vi "Read Disconnected.vi"(8 "error in (no error)":errorcluster, 11 "EventsParent in":refnum<class "Events.lvclass">) -> (0 "error out":errorcluster, 2 "Disconnected":refnum<user-event>, 3 "EventsParent out":refnum<class "Events.lvclass">)   [LabVIEW 2020, in "wamplv.lvlib" / "Events.lvclass"]
uses:
  Events.lvclass
  WAMP Client/API/TypeDefs/Disconnected event data.ctl
  WAMP Client/API/TypeDefs/Termination Reason.ctl
  WAMP Client/Private/TypeDef/Termination Reason Enum.ctl
  Events.lvclass/Events.ctl
  WAMP Client/WAMP Client.lvclass
  wamplv.lvlib
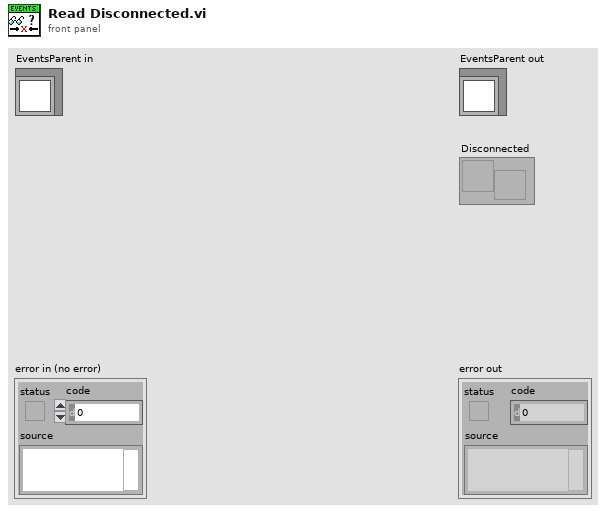
[diagram p1: front panel]
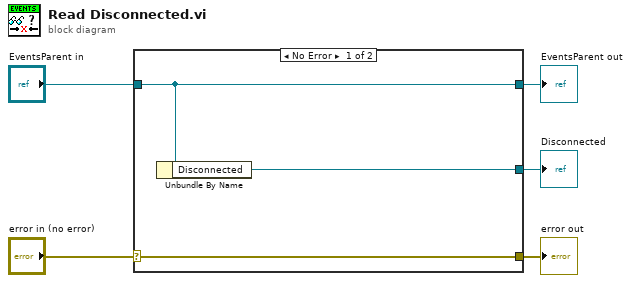
[diagram p0: block diagram]
diagram:
  n1 = case shown="No Error" "error in (no error)" {
    selector: "error in (no error)" -> [w8 w9]
    tunnel: [w8 w9] -> w4
    tunnel: [w7 w10] -> w2
    tunnel: "EventsParent in" -> [w7 w10]
    tunnel: [w6 _] -> w1
    frame No Error {
      n2 = Unbundle By Name(w7) -> ("Disconnected"=w6:refnum<user-event>)
    }
    frame Error {
    }
  }
  "error out" <- w4
  "EventsParent out" <- w2
  "Disconnected" <- w1
